vi "data analysis5 (1).vi"() -> ()   [LabVIEW 2012]
uses:
  <vilib>/Utility/file.llb/Read From Spreadsheet File (DBL).vi
  <vilib>/Utility/file.llb/Read From Spreadsheet File (string).vi
  <vilib>/Utility/file.llb/Write To Spreadsheet File (DBL).vi
  <vilib>/Analysis/NI_AALBase.lvlib
panel:
  out "x+y 2":i32
  out "String converted to Time Stamp 2":timestamp
  out "output 2":timestamp
  out "Array":timestamp[](array[timestamp])
  out "Cursor.Cursor Position:Cursor X":dbl
  out "double precision float":dbl
  in  "Ring":u16(ring) items=["Temperature", "Humidity"]
  out "x+y":i32
  out "String converted to Time Stamp":timestamp
  out "Raw Data":dbl[][](graph)
  out "Time":string[](array[string])
  out "Temp":dbl[](array[numeric])
  out "Humid":dbl[](array[numeric])
  out "Current Data":dbl[](graph)
  in  "Log data value":bool
  out "standard deviation":dbl format="%0.2f"
  out "mean":dbl format="%0.2f"
  in  "stop":bool
  out "Data Section":dbl[][](graph)
  in  "Path":path=path "C:/Users/Deely/Desktop/test.txt"
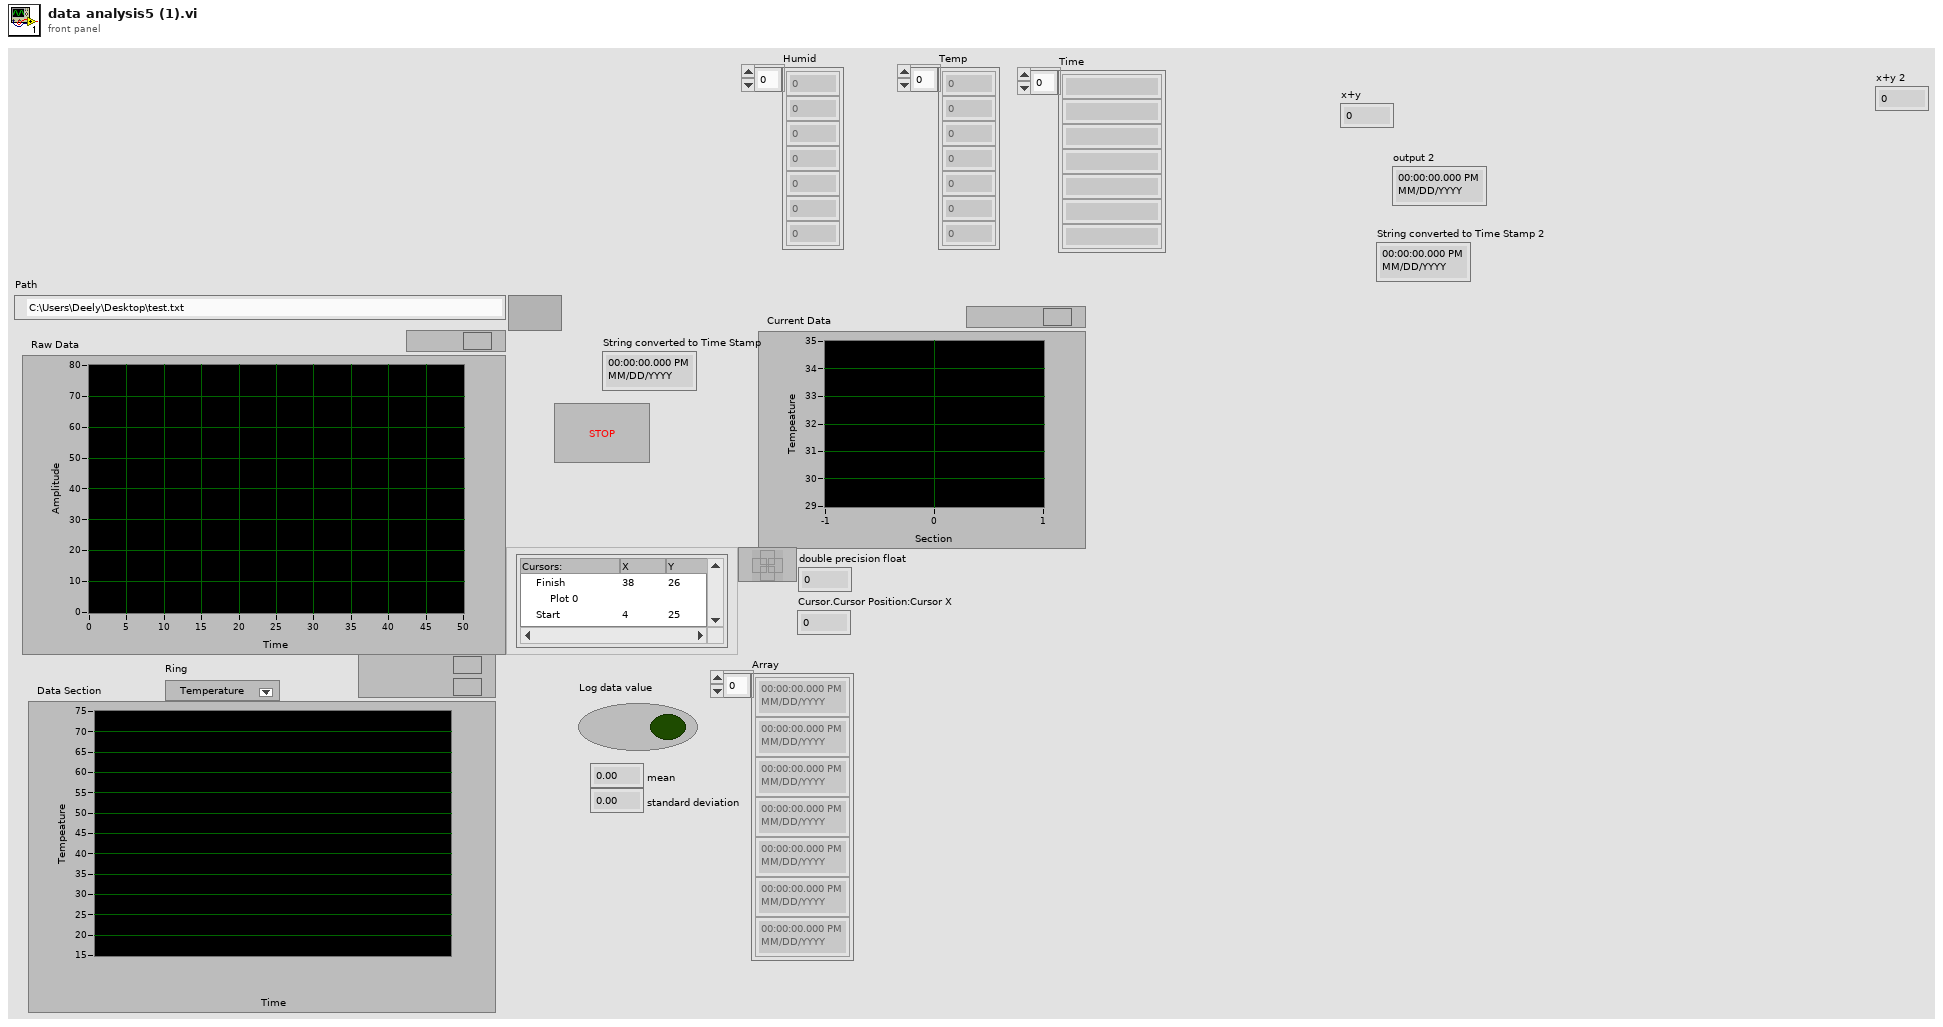
[diagram p1: front panel]
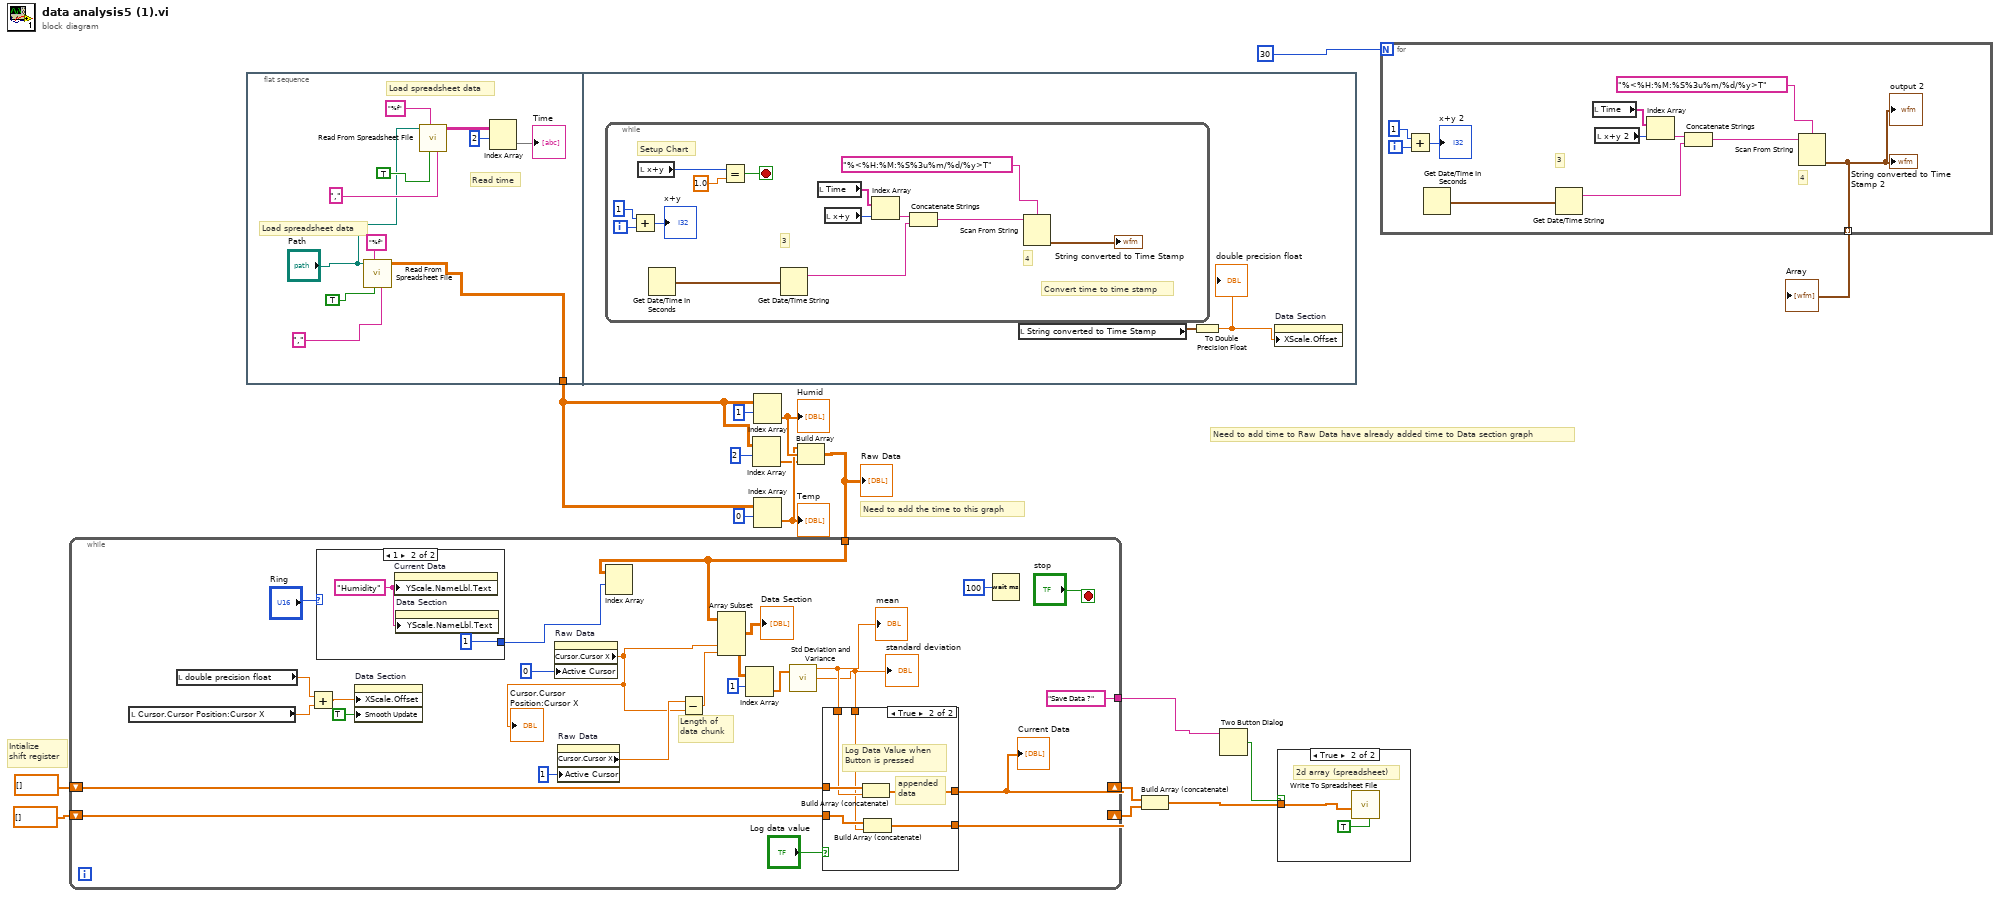
[diagram p0: block diagram]
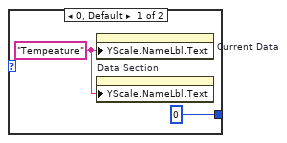
[diagram p3: hidden frame]
diagram:
  # "Need to add time to Raw Data have already added time to Data section graph"
  # "Need to add the time to this graph"
  # "Intialize \nshift register"
  n1 = flat-sequence {
    tunnel: [w19] -> w2
    frame #0 {
      # "Read time"
      # "Load spreadsheet data"
      # "Load spreadsheet data"
      n2 = call-poly <vilib>:"Read From Spreadsheet File.vi"("delimiter (\\t)"=",", "transpose (no:F)"=TRUE, "format (%.3f)"="%f", "file path (dialog if empty)"="Path") -> ("all rows"=w19:dbl[][])  [unwired: 3 in, 4 out]
      n3 = call-poly <vilib>:"Read From Spreadsheet File.vi"("delimiter (\\t)"=",", "transpose (no:F)"=TRUE, "format (%s)"="%f" ("format (%.3f)"), "file path (dialog if empty)"="Path") -> ("all rows"=w21:string[][])  [unwired: 3 in, 4 out]
      n4 = Index Array(array=w21, index (row)=2) -> (element=→"Time":string[])  [unwired: 1 in]
    }
    frame #1 {
      n5 = while {
        i -> [w32]
        stop <- w33 stop-if-true
        # "Convert time to time stamp"
        # "4"
        # "3"
        # "Setup Chart"
        n6 = Add(x=1, y=w32) -> (x+y=→"x+y":i32)
        n7 = local read "x+y"() -> (w41:i32)
        n8 = Get Date/Time In Seconds() -> (seconds since 1Jan1904=w34:timestamp)
        n9 = Equal?(x=w41, y=1.0 ("x")) -> (x = y?=w33:bool)
        n10 = Get Date/Time String(seconds (now)=w34) -> (date string=w40:string)  [unwired: 3 out]
        n11 = local read "Time"() -> (w37:string[])
        n12 = local read "x+y"() -> (w36:i32)
        n13 = Index Array(array=w37, index=w36) -> (element=w35:string)
        n14 = Concatenate Strings "Concatenate Strings"(w35, w40) -> (w39:string)
        n15 = Scan From String "Scan From String"(format string="%<%H:%M:%S%3u%m/%d/%y>T" ("input string"), input string=w39) -> (output 1=→"String converted to Time Stamp":timestamp)  [unwired: 2 in, 4 out]
      }
      n16 = local read "String converted to Time Stamp"() -> (w30:timestamp)
      n17 = To Double Precision Float(number=w30) -> (double precision float=w29:dbl)
      "double precision float" <- w29
      n18 = property on="Data Section" class="WFGraph (strict)"("XScale.Offset"=w29) -> ()  [unwired: 2 in, 2 out]
    }
  }
  n19 = Index Array(array=w2, index (row)=2) -> (element=w1:dbl[])  [unwired: 1 in]
  n20 = Index Array(array=w2, index (row)=1) -> (element=w5:dbl[])  [unwired: 1 in]
  "Humid" <- w5
  n21 = Index Array(array=w2, index (row)=0) -> (element=w4:dbl[])  [unwired: 1 in]
  "Temp" <- w4
  n22 = Build Array(w4, w5, w1) -> (w6:dbl[][])
  "Raw Data" <- w6
  n23 = while {
    shift-right: [w64] -> w14
    shift-left: dbl[] [] ("subarray") -> [w66]
    shift-right: [w61] -> w15
    shift-left: dbl[] [] ("subarray") -> [w63]
    tunnel: ["Save Data ?" ("message")] -> w11
    tunnel: w6 -> [w50]
    stop <- "stop" stop-if-true
    # "Length of \ndata chunk"
    n24 = local read "Cursor.Cursor Position:Cursor X"() -> (w52:dbl)
    n25 = local read "double precision float"() -> (w53:dbl)
    n26 = Add(x=w53, y=w52) -> (x+y=w51:dbl)
    n27 = case shown="1" "Ring" {
      tunnel: [0 ("index (row)") 1 ("index (row)")] -> w56
      frame 0, Default {
        w70 = "Tempeature" ("Y Scale.Unit Label.Text")
        n28 = property on="Current Data" class="WFGraph (strict)"("YScale.NameLbl.Text"=w70) -> ()  [unwired: 2 in, 2 out]
        n29 = property on="Data Section" class="WFGraph (strict)"("YScale.NameLbl.Text"=w70) -> ()  [unwired: 2 in, 2 out]
      }
      frame 1 {
        w72 = "Humidity" ("Y Scale.Unit Label.Text")
        n30 = property on="Current Data" class="WFGraph (strict)"("YScale.NameLbl.Text"=w72) -> ()  [unwired: 2 in, 2 out]
        n31 = property on="Data Section" class="WFGraph (strict)"("YScale.NameLbl.Text"=w72) -> ()  [unwired: 2 in, 2 out]
      }
    }
    n32 = property on="Data Section" class="WFGraph (strict)"("XScale.Offset"=w51, "Smooth Update"=TRUE) -> ()  [unwired: 2 in, 2 out]
    n33 = property on="Raw Data" class="WFGraph (strict)"("Active Cursor"=u32 0) -> ("Cursor.Cursor X"=w49:dbl)  [unwired: 2 in, 2 out]
    "Cursor.Cursor Position:Cursor X" <- w49
    n34 = property on="Raw Data" class="WFGraph (strict)"("Active Cursor"=u32 1) -> ("Cursor.Cursor X"=w55:dbl)  [unwired: 2 in, 2 out]
    n35 = Index Array(array=w50, index (row)=w56) -> ()  [unwired: 1 in, 1 out]
    n36 = Subtract(x=w55, y=w49) -> (x-y=w48:dbl)
    n37 = Array Subset(array=w50, index (col)=w49, length (col)=w48) -> (w47:dbl[][])  [unwired: 2 in]
    "Data Section" <- w47
    n38 = Index Array(array=w47, index (row)=1) -> (element=w46:dbl[])  [unwired: 1 in]
    n39 = call <vilib>:"Std Deviation and Variance.vi"("X"=w46) -> ("mean"=w65:dbl, "standard deviation"=w62:dbl)  [unwired: 1 in, 1 out]
    "mean" <- w65
    "standard deviation" <- w62
    n40 = case shown="True" "Log data value" {
      tunnel: w66 -> [w75 w81]
      tunnel: w65 -> [_ w80]
      tunnel: [w75 w79] -> w64
      tunnel: w63 -> [w74 w78]
      tunnel: w62 -> [_ w77]
      tunnel: [w74 w76] -> w61
      frame False {
        # "Do nothing just pass\n data through"
      }
      frame True {
        # "appended\ndata"
        # "Log Data Value when \nButton is pressed"
        n41 = Build Array (concatenate)(w81, w80) -> (w79:dbl[])
        n42 = Build Array (concatenate)(w78, w77) -> (w76:dbl[])
      }
    }
    "Current Data" <- w64
    n43 = Wait (ms)(milliseconds to wait=u32 100) -> ()  [unwired: 1 out]
  }
  n44 = Build Array (concatenate)(w14, w15) -> (w13:dbl[])
  n45 = Two Button Dialog(message=w11) -> (T button?=w12:bool)  [unwired: 2 in]
  n46 = case shown="True" w12 {
    tunnel: w13 -> [_ w83]
    frame False {
    }
    frame True {
      # "2d array (spreadsheet)"
      n47 = call-poly <vilib>:"Write To Spreadsheet File.vi"("transpose? (no:F)"=TRUE, "1D data"=w83) -> ()  [unwired: 6 in, 1 out]
    }
  }
  n48 = for {
    N: 30 -> [_]
    tunnel: [w84] -> w7 mode=indexing
    i -> [w85]
    # "4"
    # "3"
    n49 = Add(x=1, y=w85) -> (x+y=→"x+y 2":i32)
    n50 = Get Date/Time In Seconds() -> (seconds since 1Jan1904=w86:timestamp)
    n51 = Get Date/Time String(seconds (now)=w86) -> (date string=w92:string)  [unwired: 3 out]
    n52 = local read "Time"() -> (w89:string[])
    n53 = local read "x+y 2"() -> (w88:i32)
    n54 = Index Array(array=w89, index=w88) -> (element=w87:string)
    n55 = Concatenate Strings "Concatenate Strings"(w87, w92) -> (w91:string)
    n56 = Scan From String "Scan From String"(format string="%<%H:%M:%S%3u%m/%d/%y>T" ("input string"), input string=w91) -> (output 1=w84:timestamp)  [unwired: 2 in, 4 out]
    "String converted to Time Stamp 2" <- w84
    "output 2" <- w84
  }
  "Array" <- w7
